vi "Read Async Methods Running Event Ref.vi"(8 "error in (no error)":errorcluster, 11 "Async Methods Actor in":refnum<class "Async Methods Actor.lvclass">) -> (0 "error out":errorcluster, 2 "Async Methods Running Event Ref":refnum<user-event>, 3 "Async Methods Actor out":refnum<class "Async Methods Actor.lvclass">)   [LabVIEW 2021, in "Async Methods Actor.lvlib" / "Async Methods Actor.lvclass"]
uses:
  Async Methods Actor.lvclass
  Async Methods Actor.lvclass/Async Methods Actor.ctl
  Async Methods Running.ctl
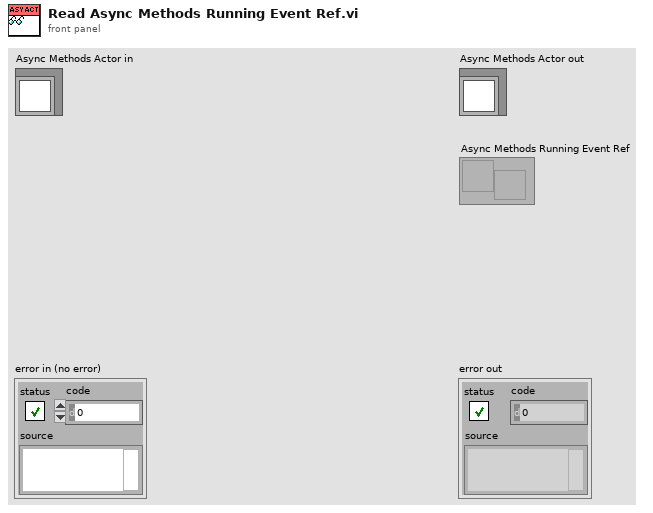
[diagram p1: front panel]
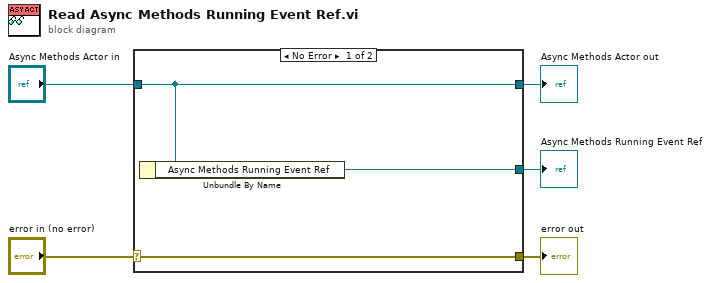
[diagram p0: block diagram]
diagram:
  n1 = case shown="No Error" "error in (no error)" {
    selector: "error in (no error)" -> [w8 w9]
    tunnel: [w8 w9] -> w4
    tunnel: [w7 w10] -> w2
    tunnel: "Async Methods Actor in" -> [w7 w10]
    tunnel: [w6 _] -> w1
    frame No Error {
      n2 = Unbundle By Name(w7) -> ("Async Methods Running Event Ref"=w6:refnum<user-event>)
    }
    frame Error {
    }
  }
  "error out" <- w4
  "Async Methods Actor out" <- w2
  "Async Methods Running Event Ref" <- w1
